vi "Sandbox.vi"() -> ()   [LabVIEW 2019, in "OWEN HMI.lvclass"]
uses:
  OWEN HMI.lvclass
  Bit.ctl
  Words.ctl
  19f3744f-72bc-4c39-aaca-5bdf827a74e4.vi
  b80abefe-0104-4203-839a-19dc6cb4a819.vi
  Global - Data.vi
panel:
  in  "stop":bool
  out "error out":errorcluster
  in  "error in":errorcluster
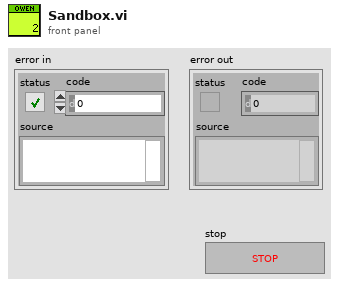
[diagram p1: front panel]
types:
  T1 = typedef "OWEN HMI.lvclass/Bit.ctl" = enum16{"0 - Pump CC", "1 - Pump SO", "2 - Alarm", "3 - Warning", "4 - DUT", "5 - CHMBR"}
  T2 = typedef "OWEN HMI.lvclass/Words.ctl" = enum16{"0 - Bits", "1 - Level CC", "2 - Temp CC", "3 - Level SO", "4 - Temp SO"}
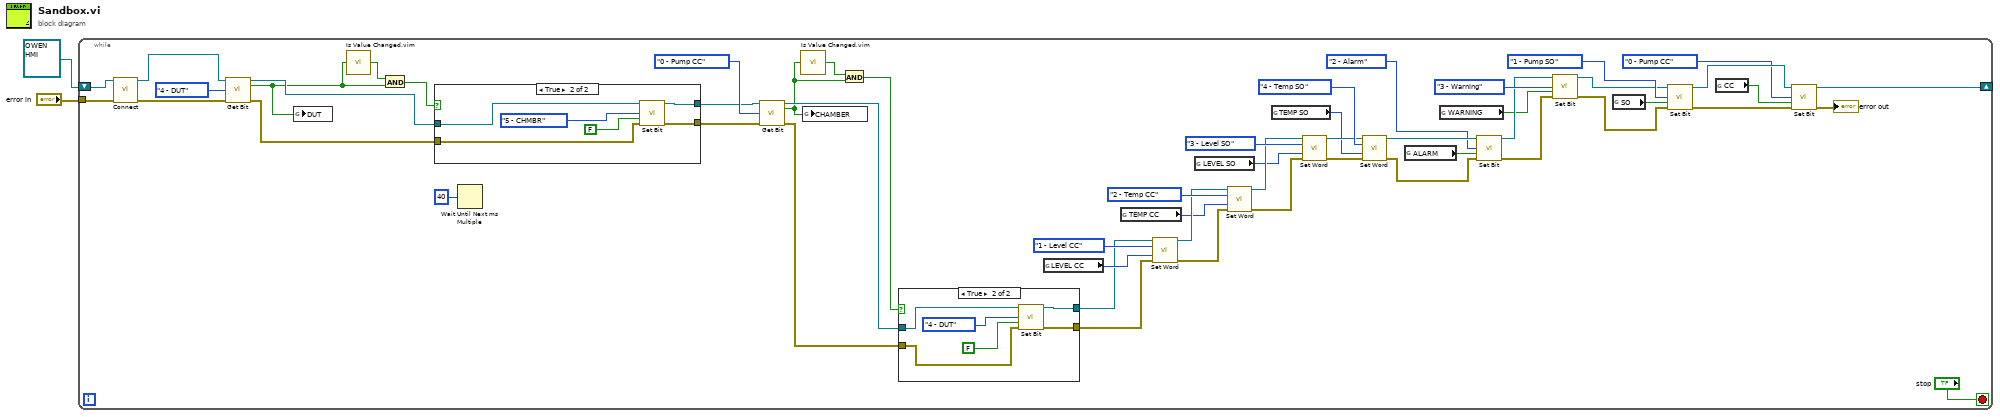
[diagram p0: block diagram]
diagram:
  n1 = while {
    tunnel: "error in" -> [w56]
    shift-right: [w4] -> _
    shift-left: refnum<class "OWEN HMI.lvclass"> refnum ("OWEN HMI.lvclass") -> [w28]
    stop <- "stop" stop-if-true
    n2 = call "Connect.vi"("OWEN HMI in"=w28, "error in (no error)"=w56) -> ("OWEN HMI out"=w55:refnum<class "OWEN HMI.lvclass">, "error out"=w54:errorcluster)  [unwired: 12 in]
    n3 = call "Get Bit.vi"("OWEN HMI in"=w55, "bit"=Bit."4 - DUT", "error in (no error)"=w54) -> ("OWEN HMI out"=w53:refnum<class "OWEN HMI.lvclass">, "value"=w20:bool, "error out"=w52:errorcluster)  [unwired: 10 in]
    n4 = global write "Global - Data.vi" "DUT"(w20) -> ()
    n5 = call "Is Value Changed.vim"("value"=w20) -> ("changed or first call?"=w19:bool)
    n6 = And(x=w19, y=w20) -> (x .and. y?=w50:bool)
    n7 = case shown="True" w50 {
      tunnel: w53 -> [w66 w72]
      tunnel: w52 -> [w65 w71]
      tunnel: [w66 w69] -> w18
      tunnel: [w65 w68] -> w17
      frame False {
      }
      frame True {
        n8 = call "Set Bit.vi"("OWEN HMI in"=w72, "bit"=Bit."5 - CHMBR", "value"=FALSE, "error in (no error)"=w71) -> ("OWEN HMI out"=w69:refnum<class "OWEN HMI.lvclass">, "error out"=w68:errorcluster)  [unwired: 10 in]
      }
    }
    n9 = Wait Until Next ms Multiple(millisecond multiple=u32 40 ("milliseconds to wait")) -> ()  [unwired: 1 out]
    n10 = call "Get Bit.vi"("OWEN HMI in"=w18, "bit"=Bit."0 - Pump CC", "error in (no error)"=w17) -> ("OWEN HMI out"=w47:refnum<class "OWEN HMI.lvclass">, "value"=w14:bool, "error out"=w48:errorcluster)  [unwired: 10 in]
    n11 = call "Is Value Changed.vim"("value"=w14) -> ("changed or first call?"=w15:bool)
    n12 = global write "Global - Data.vi" "CHAMBER"(w14) -> ()
    n13 = And(x=w15, y=w14) -> (x .and. y?=w49:bool)
    n14 = case shown="True" w49 {
      tunnel: w47 -> [w58 w64]
      tunnel: w48 -> [w57 w63]
      tunnel: [w58 w61] -> w16
      tunnel: [w57 w60] -> w13
      frame False {
      }
      frame True {
        n15 = call "Set Bit.vi"("OWEN HMI in"=w64, "bit"=Bit."4 - DUT", "value"=FALSE, "error in (no error)"=w63) -> ("OWEN HMI out"=w61:refnum<class "OWEN HMI.lvclass">, "error out"=w60:errorcluster)  [unwired: 10 in]
      }
    }
    n16 = global read "Global - Data.vi" "LEVEL CC"() -> (w22:i16)
    n17 = global read "Global - Data.vi" "TEMP CC"() -> (w23:i16)
    n18 = call "Set Word.vi"("OWEN HMI in"=w16, "address"=Words."1 - Level CC", "value"=w22, "error in (no error)"=w13) -> ("OWEN HMI out"=w44:refnum<class "OWEN HMI.lvclass">, "error out"=w43:errorcluster)  [unwired: 10 in]
    n19 = global read "Global - Data.vi" "LEVEL SO"() -> (w24:i16)
    n20 = call "Set Word.vi"("OWEN HMI in"=w44, "address"=Words."2 - Temp CC", "value"=w23, "error in (no error)"=w43) -> ("OWEN HMI out"=w41:refnum<class "OWEN HMI.lvclass">, "error out"=w40:errorcluster)  [unwired: 10 in]
    n21 = global read "Global - Data.vi" "TEMP SO"() -> (w25:i16)
    n22 = call "Set Word.vi"("OWEN HMI in"=w41, "address"=Words."3 - Level SO", "value"=w24, "error in (no error)"=w40) -> ("OWEN HMI out"=w38:refnum<class "OWEN HMI.lvclass">, "error out"=w37:errorcluster)  [unwired: 10 in]
    n23 = call "Set Word.vi"("OWEN HMI in"=w38, "address"=Words."4 - Temp SO", "value"=w25, "error in (no error)"=w37) -> ("OWEN HMI out"=w36:refnum<class "OWEN HMI.lvclass">, "error out"=w35:errorcluster)  [unwired: 10 in]
    n24 = global read "Global - Data.vi" "ALARM"() -> (w27:bool)
    n25 = global read "Global - Data.vi" "WARNING"() -> (w26:bool)
    n26 = call "Set Bit.vi"("OWEN HMI in"=w36, "bit"=Bit."2 - Alarm", "value"=w27, "error in (no error)"=w35) -> ("OWEN HMI out"=w32:refnum<class "OWEN HMI.lvclass">, "error out"=w31:errorcluster)  [unwired: 10 in]
    n27 = call "Set Bit.vi"("OWEN HMI in"=w32, "bit"=Bit."3 - Warning", "value"=w26, "error in (no error)"=w31) -> ("OWEN HMI out"=w5:refnum<class "OWEN HMI.lvclass">, "error out"=w6:errorcluster)  [unwired: 10 in]
    n28 = global read "Global - Data.vi" "SO"() -> (w11:bool)
    n29 = call "Set Bit.vi"("OWEN HMI in"=w5, "bit"=Bit."1 - Pump SO", "value"=w11, "error in (no error)"=w6) -> ("OWEN HMI out"=w9:refnum<class "OWEN HMI.lvclass">, "error out"=w10:errorcluster)  [unwired: 10 in]
    n30 = global read "Global - Data.vi" "CC"() -> (w12:bool)
    n31 = call "Set Bit.vi"("OWEN HMI in"=w9, "bit"=Bit."0 - Pump CC", "value"=w12, "error in (no error)"=w10) -> ("OWEN HMI out"=w4:refnum<class "OWEN HMI.lvclass">, "error out"=→"error out":errorcluster)  [unwired: 10 in]
  }
